vi "py-lv-comm_callFunction.vi"(6 "Wait for response (T)":bool=TRUE, 7 "Property (F)":bool, 8 "error in (no error)":errorcluster, 9 "arguments":string[](array[string]), 10 "function":string, 11 "zmq_socket in":refnum<class "zmq_socket.lvclass">=refnum) -> (0 "error out":errorcluster, 2 "return value":string, 3 "zmq_socket out":refnum<class "zmq_socket.lvclass">)   [LabVIEW 2016]
doc: "Calls a function via the ZMQ socket.\nIf \"Wait for response\" is False, the function will immediately return after sending. The data string will then be empty.\nIn case \"Wait for response\" is True, the function will block until a message is received on the socket.\nThe \"arguments\" array is an array of strings. All elements of the array are passed to the function as arguments.\n\nIf \"Property\" == True, the \"function\" is called without any arguments and without\nthe brackets => Access to a python @property."
uses:
  <vilib>/addons/zeromq/zmq_socket.lvclass
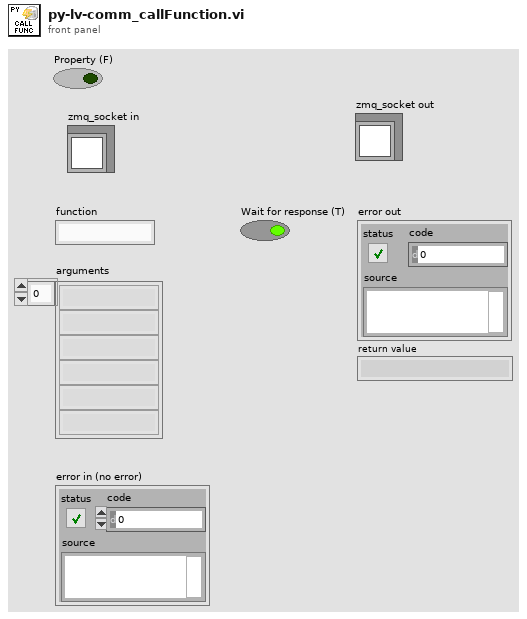
[diagram p1: front panel]
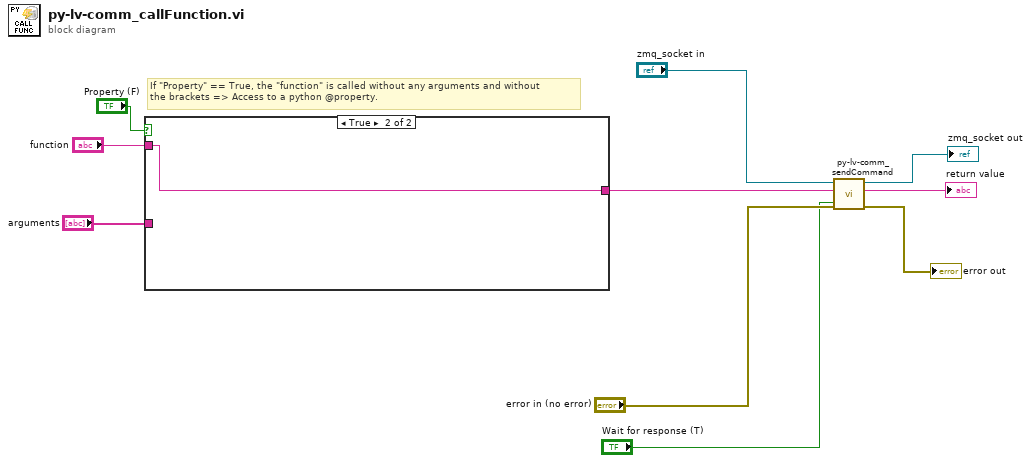
[diagram p0: block diagram]
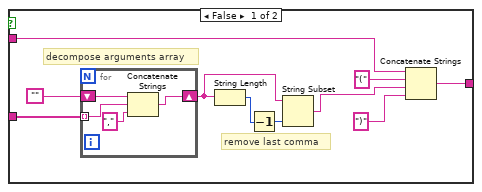
[diagram p2: hidden frame]
diagram:
  # "If \"Property\" == True, the \"function\" is called without any arguments and without\nthe brackets => Access to a python @property."
  n1 = case shown="True" "Property (F)" {
    tunnel: [w18 w25] -> w10
    tunnel: "arguments" -> [w12 _]
    tunnel: "function" -> [w11 w25]
    frame False {
      # "remove last comma"
      # "decompose arguments array"
      n2 = for {
        tunnel: w12 -> [w23] mode=indexing
        shift-right: [w21] -> w14
        shift-left: "" -> [w24]
        n3 = Concatenate Strings(w24, w23, "," ("string")) -> (w21:string)
      }
      n4 = String Length(string=w14) -> (length=w16:i32)
      n5 = Decrement(x=w16) -> (x-1=w15:i32)
      n6 = String Subset(string=w14, length (rest)=w15) -> (substring=w13:string)  [unwired: 1 in]
      n7 = Concatenate Strings(w11, "(" ("string"), w13, ")" ("string")) -> (w18:string)
    }
    frame True {
    }
  }
  n8 = call "py-lv-comm_sendCommand.vi"("Wait for response (T)"="Wait for response (T)", "error in (no error)"="error in (no error)", "command"=w10, "zmq_socket in"="zmq_socket in") -> ("error out"=→"error out":errorcluster, "data"=→"return value":string, "zmq_socket out"=→"zmq_socket out":refnum<class "zmq_socket.lvclass">)  [unwired: 5 in]
